vi "Extract Channel Information.vi"(11 "Channel Info File":path) -> (2 "Pin Info List":T2, 3 "Channel List":T4)   [LabVIEW 2021]
uses:
  <vilib>/myRIO/Common/Instrument Driver Framework/Utilities/typedefs/Channel List Array.ctl
  <vilib>/myRIO/Common/Instrument Driver Framework/Utilities/typedefs/Channel List Cluster.ctl
  <vilib>/myRIO/Common/Instrument Driver Framework/Utilities/typedefs/Pin Info List Array.ctl
  <vilib>/myRIO/Common/Instrument Driver Framework/Utilities/typedefs/Pin Info Cluster.ctl
  <vilib>/myRIO/Common/Instrument Driver Framework/Utilities/typedefs/Channel Types.ctl
  <vilib>/myRIO/Common/FPGA Personality Framework/Personality.lvlib
panel:
  in  "Channel Types":T1
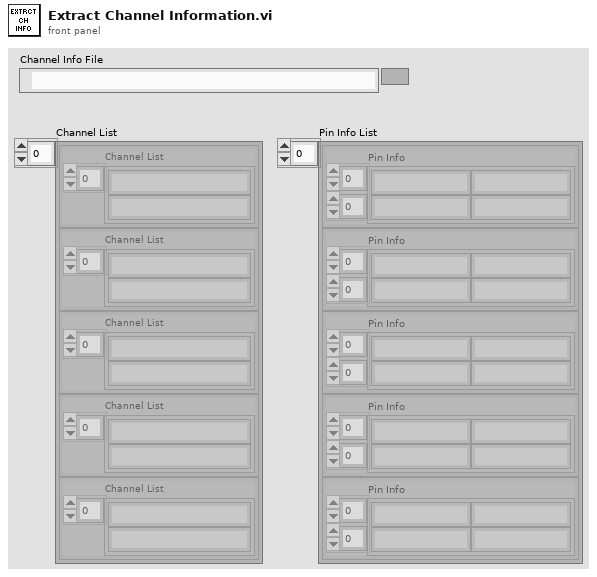
[diagram p1: front panel]
types:
  T1 = typedef "Channel Types.ctl" = enum32{"Unknown", "AI", "AO", "DIO - DI", "DIO", "DIO - DO", "I2C", "PWM", "Encoder", "SPI", "UART", "Accelerometer", "DIO - LED", "DIO - Button", "AI (N Samples)", "AudioIn (N Samples)", "AO (N Samples)", "AudioOut (N Samples)", "DI (N Samples)", "DO (N Samples)", "AI IRQ", "DI IRQ", "Timer IRQ", "RSL", "Relay", "CAN", "AI (Continuous)", "AO (Continuous)"}
  T2 = typedef "Pin Info List Array.ctl" = T3[]
  T3 = typedef "Pin Info Cluster.ctl" = cluster{"Pin Info":string[][]}
  T4 = typedef "Channel List Array.ctl" = T5[]
  T5 = typedef "Channel List Cluster.ctl" = cluster{"Channel List":string[]}
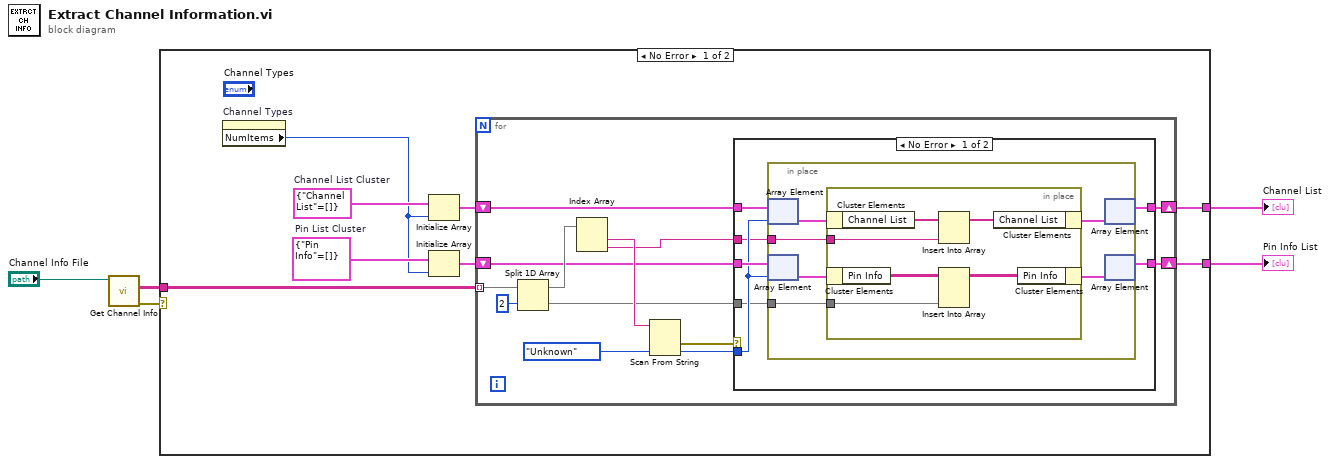
[diagram p0: block diagram]
diagram:
  n1 = call <vilib>:"Get Channel Info.vi"("FPGA Personality File Path"="Channel Info File") -> ("error out"=w3:errorcluster, "Channel Info"=w1:string[][])  [unwired: 8 in, 1 out]
  n2 = case shown="No Error" w3 {
    tunnel: [w10 _] -> w5
    tunnel: [w9 _] -> w4
    tunnel: w1 -> [w6 _]
    frame No Error {
      w8 = T5 {"Channel List"=[]}  # Channel List Cluster
      w13 = T3 {"Pin Info"=[]}  # Pin List Cluster
      n3 = property on="Channel Types" class="Enum (strict)"() -> ("NumItems"=w7:u32)  [unwired: 2 in, 2 out]
      n4 = Initialize Array(w8, w7) -> (w12:T5[])
      n5 = Initialize Array(w13, w7) -> (w11:T3[])
      n6 = for {
        tunnel: w6 -> [w26] mode=indexing
        shift-right: [w19] -> w10
        shift-left: w12 -> [w22]
        shift-right: [w18] -> w9
        shift-left: w11 -> [w21]
        n7 = Split 1D Array(array=w26, index=2) -> (first subarray=w24:string[], second subarray=w16:string[])
        n8 = Index Array(array=w24) -> (element #1=w23:string, element #2=w17:string)  [unwired: 2 in]
        n9 = Scan From String(input string=w23, default 1=Channel_Types."Unknown" ("Channel Types")) -> (error out=w14:errorcluster, output 1=w20:T1)  [unwired: 3 in, 2 out]
        n10 = case shown="No Error" w14 {
          tunnel: w22 -> [w33 w47]
          tunnel: w21 -> [w32 w46]
          tunnel: w20 -> [w31 _]
          tunnel: [w30 w47] -> w19
          tunnel: [w29 w46] -> w18
          tunnel: w17 -> [w28 _]
          tunnel: w16 -> [w27 _]
          frame No Error {
            n11 = in-place {
              in-place-border: w28 -> [w38]
              in-place-border: w27 -> [w35]
              n12 = in-place-array #1(w33, w31) -> (w39:T5)
              n13 = in-place-array #2(w32, w31) -> (w36:T3)
              n14 = in-place {
                in-place-border: w38 -> [w43]
                in-place-border: w35 -> [w40]
                n15 = in-place-cluster #3(w39) -> ("Channel List"=w45:string[])
                n16 = in-place-cluster #4(w36) -> ("Pin Info"=w42:string[][])
                n17 = Insert Into Array(array=w45, new element=w43) -> (w44:string[])  [unwired: 1 in]
                n18 = Insert Into Array(array=w42, new element=w40) -> (w41:string[][])  [unwired: 2 in]
                n19 = in-place-cluster #3("Channel List"=w44) -> (w37:T5)
                n20 = in-place-cluster #4("Pin Info"=w41) -> (w34:T3)
              }
              n21 = in-place-array #1(w37) -> (w30:T5[])  [unwired: 1 out]
              n22 = in-place-array #2(w34) -> (w29:T3[])  [unwired: 1 out]
            }
          }
          frame Error {
          }
        }
      }
    }
    frame Error {
    }
  }
  "Channel List" <- w5
  "Pin Info List" <- w4
